vi "Gaussian Kernel.vi"(11 "radius":u16) -> (0 "1/2 Kernel size":u16, 3 "Kernel":dbl[](graph))   [LabVIEW 2018]
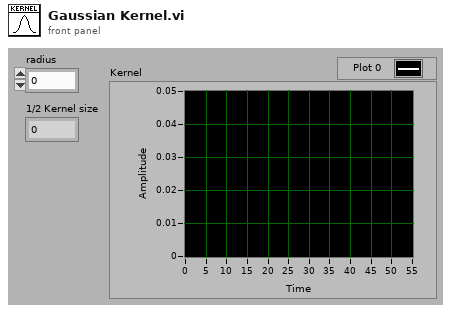
[diagram p1: front panel]
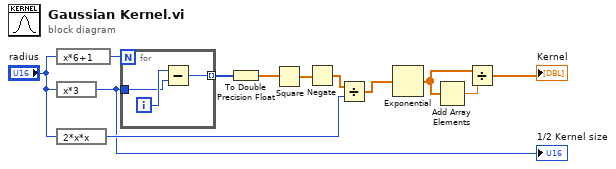
[diagram p0: block diagram]
diagram:
  n1 = expression code="x*6+1"("radius") -> (w12:u16)
  n2 = expression code="x*3"("radius") -> (w1:u16)
  "1/2 Kernel size" <- w1
  n3 = expression code="2*x*x"("radius") -> (w7:u16)
  n4 = for {
    N: w12 -> [_]
    tunnel: [w14] -> w11 mode=indexing
    tunnel: w1 -> [w13]
    i -> [w15]
    n5 = Subtract(x=w15, y=w13) -> (x-y=w14:i32)
  }
  n6 = To Double Precision Float(number=w11) -> (double precision float=w10:dbl[])
  n7 = Square(x=w10) -> (x^2=w9:dbl[])
  n8 = Negate(x=w9) -> (-x=w8:dbl[])
  n9 = Divide(x=w8, y=w7) -> (x/y=w6:dbl[])
  n10 = Exponential(1:w6) -> (0:w5:dbl[])
  n11 = Add Array Elements(numeric array=w5) -> (sum=w4:dbl)
  n12 = Divide(x=w5, y=w4) -> (x/y=→"Kernel":dbl[])
